vi "PostLoop.vi"(6 "Error":errorcluster, 7 "Actor":refnum<class "Actor.lvclass">, 10 "EventRef":refnum<event-registration>, 11 "Actor":T1) -> (3 "Actor":T1, 5 "Actor":refnum<class "Actor.lvclass">)   [LabVIEW 2020, in "jettl.lvlib"]
uses:
  jettl.lvlib
  Actor/Actor.lvclass
  Metadata/Metadata.lvclass
  Msg/Msg.lvclass
  Msg.ctl
  Origin.ctl
  Lifecycle.ctl
  MsgAttribs.ctl
  MsgExecuteType.ctl
  PostSetup.ctl
  PreSetup.ctl
  MsgNames.ctl
  ActorAttribs.ctl
  ChildActors.ctl
  Actor.ctl
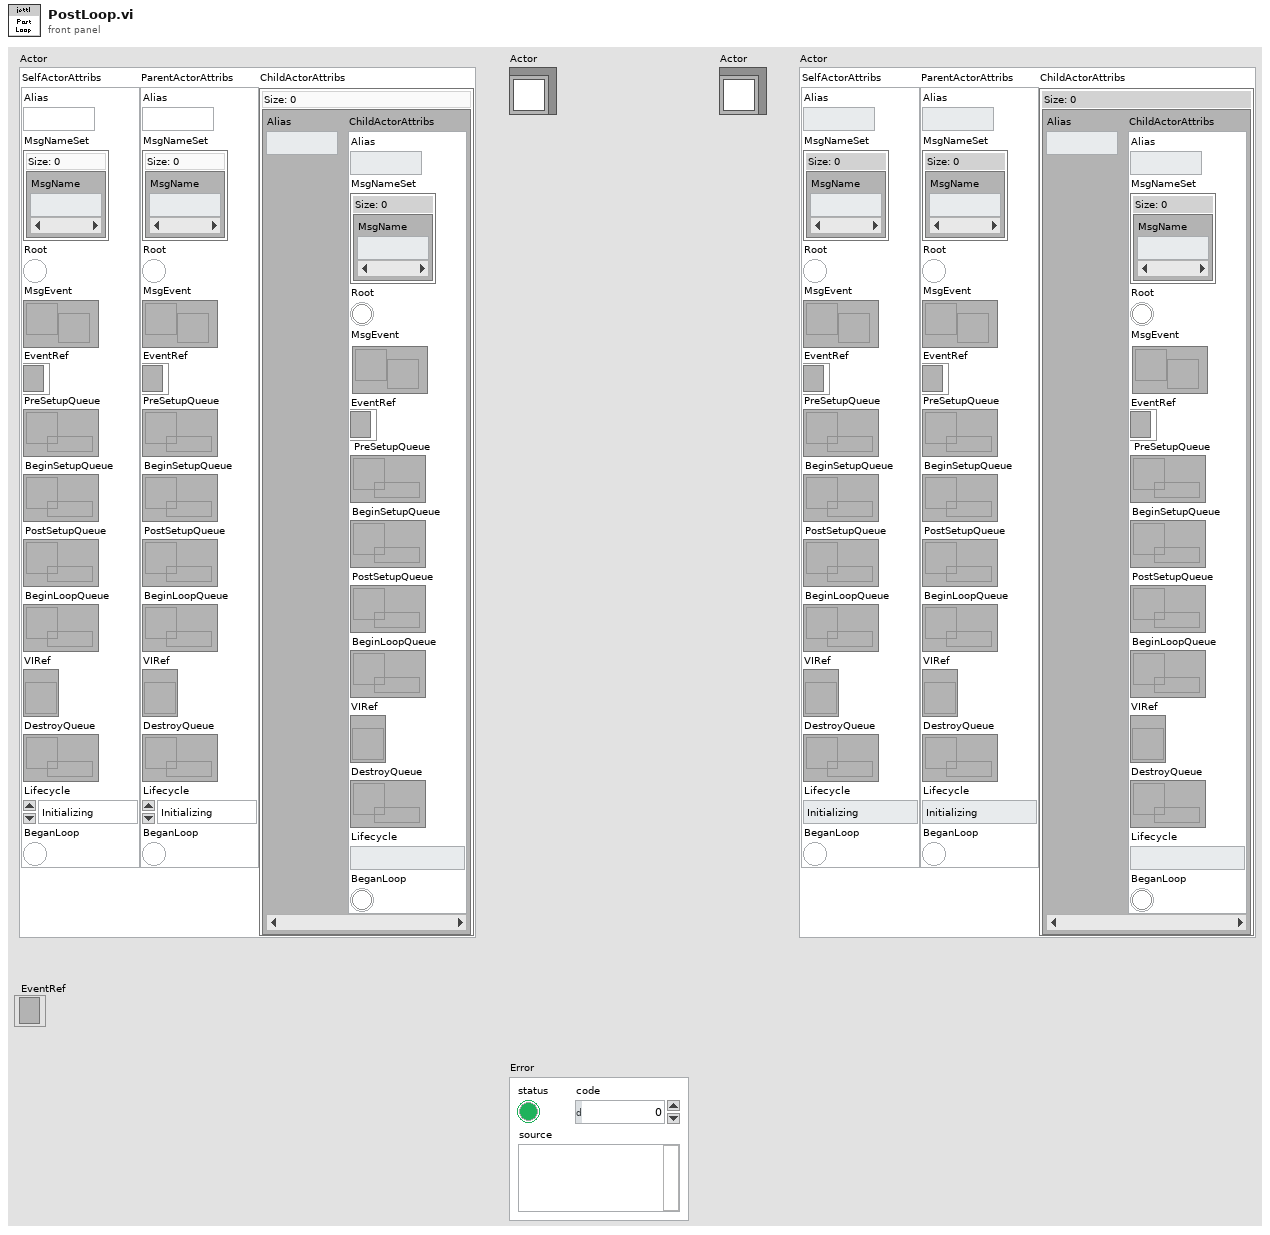
[diagram p1: front panel]
types:
  T1 = typedef "jettl.lvlib/Actor.ctl" = cluster{"SelfActorAttribs":T2, "ParentActorAttribs":T2, "ChildActorAttribs":T5}
  T2 = typedef "jettl.lvlib/ActorAttribs.ctl" = cluster{"Alias":string, "MsgNameSet":T3, "Root":bool, "MsgEvent":refnum<user-event>, "EventRef":refnum<event-registration>, "PreSetupQueue":refnum<queue>, "BeginSetupQueue":refnum<queue>, "PostSetupQueue":refnum<queue>, "BeginLoopQueue":refnum<queue>, "VIRef":refnum<vi>, "DestroyQueue":refnum<queue>, "Lifecycle":T4, "BeganLoop":bool}
  T3 = typedef "jettl.lvlib/MsgNames.ctl" = set{string}
  T4 = typedef "jettl.lvlib/Lifecycle.ctl" = enum16{"Initializing", "SettingUp", "Starting", "Running", "Stopping", "TearingDown", "Terminated"}
  T5 = typedef "jettl.lvlib/ChildActors.ctl" = map{string, T2}
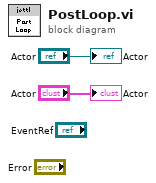
[diagram p0: block diagram]
diagram:
  "Actor" <- "Actor"
  "Actor" <- "Actor"
